vi "timestamptest.vi"() -> ()   [LabVIEW 2012]
panel:
  out "int0":i16
  out "unsigned 16bit integer":u16 format="%b"
  out "unsigned 64bit integer":u64 format="%b"
  out "x << y":u32 format="%b"
  out "x = y?":bool
  out "timestamp?":u64
  out "int3":i16
  out "int2":i16
  out "int1":i16
  in  "Numeric":u64
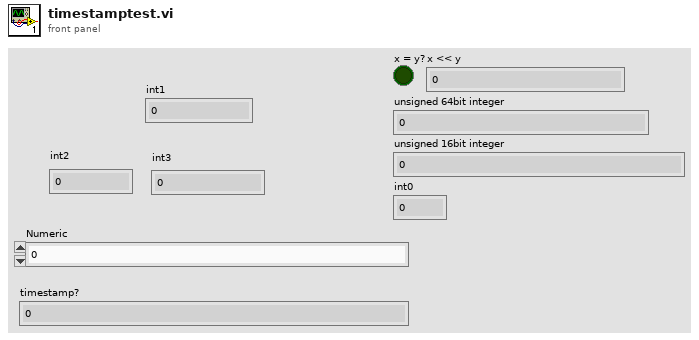
[diagram p1: front panel]
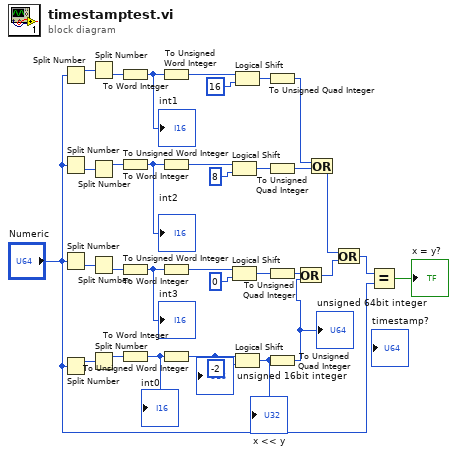
[diagram p0: block diagram]
diagram:
  n1 = Split Number(x="Numeric") -> (hi(x)=w32:u32)  [unwired: 1 out]
  n2 = Split Number(x="Numeric") -> (lo(x)=w31:u32)  [unwired: 1 out]
  n3 = Split Number(x="Numeric") -> (lo(x)=w30:u32)  [unwired: 1 out]
  n4 = Split Number(x="Numeric") -> (hi(x)=w33:u32)  [unwired: 1 out]
  n5 = Split Number(x=w32) -> (lo(x)=w12:u16)  [unwired: 1 out]
  n6 = Split Number(x=w31) -> (hi(x)=w28:u16)  [unwired: 1 out]
  n7 = Split Number(x=w30) -> (lo(x)=w27:u16)  [unwired: 1 out]
  n8 = Split Number(x=w33) -> (hi(x)=w29:u16)  [unwired: 1 out]
  n9 = To Word Integer(number=w12) -> (16bit integer=w20:i16)
  "int1" <- w20
  n10 = To Word Integer(number=w28) -> (16bit integer=w18:i16)
  "int2" <- w18
  n11 = To Word Integer(number=w27) -> (16bit integer=w16:i16)
  "int3" <- w16
  n12 = To Word Integer(number=w29) -> (16bit integer=w14:i16)
  "int0" <- w14
  n13 = To Unsigned Word Integer(number=w20) -> (unsigned 16bit integer=w19:u16)
  n14 = To Unsigned Word Integer(number=w18) -> (unsigned 16bit integer=w17:u16)
  n15 = To Unsigned Word Integer(number=w16) -> (unsigned 16bit integer=w15:u16)
  n16 = To Unsigned Word Integer(number=w14) -> (unsigned 16bit integer=w13:u16)
  "unsigned 16bit integer" <- w13
  n17 = Logical Shift(y=w17, x=u32 8) -> (x << y=w10:u32)
  n18 = Logical Shift(y=w15, x=u32 0) -> (x << y=w9:u32)
  n19 = Logical Shift(y=w19, x=u32 16) -> (x << y=w11:u32)
  n20 = Logical Shift(y=w13, x=-2) -> (x << y=w8:i32)
  "x << y" <- w8
  n21 = To Unsigned Quad Integer(1:w11) -> (0:w6:u64)
  n22 = To Unsigned Quad Integer(1:w10) -> (0:w7:u64)
  n23 = To Unsigned Quad Integer(1:w9) -> (0:w5:u64)
  n24 = To Unsigned Quad Integer(1:w8) -> (0:w4:u64)
  "unsigned 64bit integer" <- w4
  n25 = Or(x=w5, y=w4) -> (x .or. y?=w2:u64)
  n26 = Or(x=w6, y=w7) -> (x .or. y?=w3:u64)
  n27 = Or(x=w3, y=w2) -> (x .or. y?=w1:u64)
  n28 = Equal?(x=w1, y="Numeric") -> (x = y?=→"x = y?":bool)
